vi "IPS Initialize.vi"(8 "Error In":errorcluster={"status"=FALSE, "code"=1073676294, "source"=""}, 10 "Numeric":u32, 11 "VISA resource name (COM Port of Prologix Device)":refnum<visa-resource-name>="GPIB1::25::INSTR") -> ()   [LabVIEW 2013]
panel:
  out "Error Out":errorcluster={"status"=TRUE, "code"=-1073807339, "source"="VISA Read in NI USB GPIB Command.vi"}
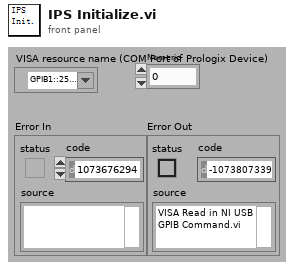
[diagram p1: front panel]
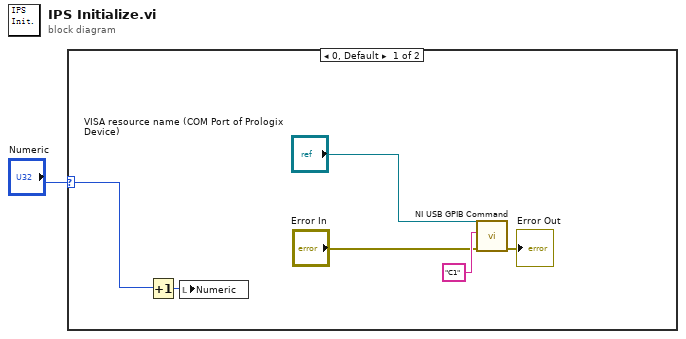
[diagram p0: block diagram]
diagram:
  n1 = case shown="0, Default" "Numeric" {
    selector: "Numeric" -> [w6 _]
    frame 0, Default {
      n2 = Increment(x=w6) -> (x+1=w5:u32)
      n3 = local write "Numeric"(w5) -> ()
      n4 = call "NI USB GPIB Command.vi"("Error In"="Error In", "String to Send"="C1", "VISA resource name"="VISA resource name (COM Port of Prologix Device)") -> ("Error Out"=→"Error Out":errorcluster)  [unwired: 1 in, 3 out]
    }
    frame 1 {
    }
  }
